vi "NameCheck.vi"(8 "error in (no error)":errorcluster, 10 "Name":string, 11 "VariableManager in":refnum<class "VariableManager.lvclass">) -> (0 "error out":errorcluster, 1 "UsedAsSequenceIndex":bool, 2 "UsedAsVariable":bool, 3 "VariableManager out":refnum<class "VariableManager.lvclass">)   [LabVIEW 2013, in "VariableManager.lvclass"]
doc: "Check the given Name agains database if it is used as a variable name or as a sequence index name (<B>idx</B>, <B>idx_f</B>, <B>idx_max</B>)."
uses:
  VariableManager.lvclass
  SequenceIndex/SequenceIndex.lvclass
  Variable/Variable.lvclass
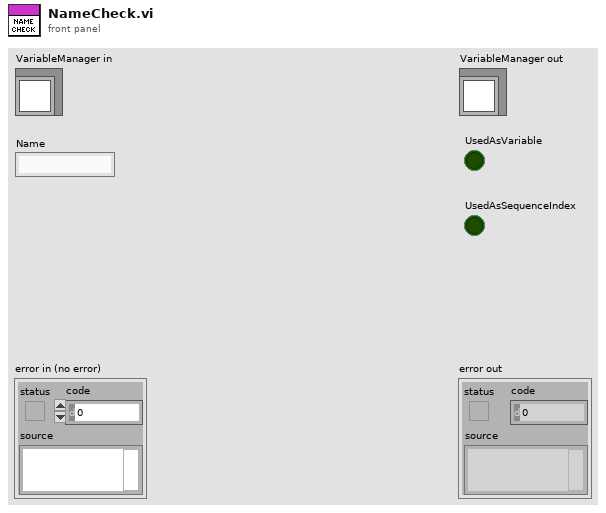
[diagram p1: front panel]
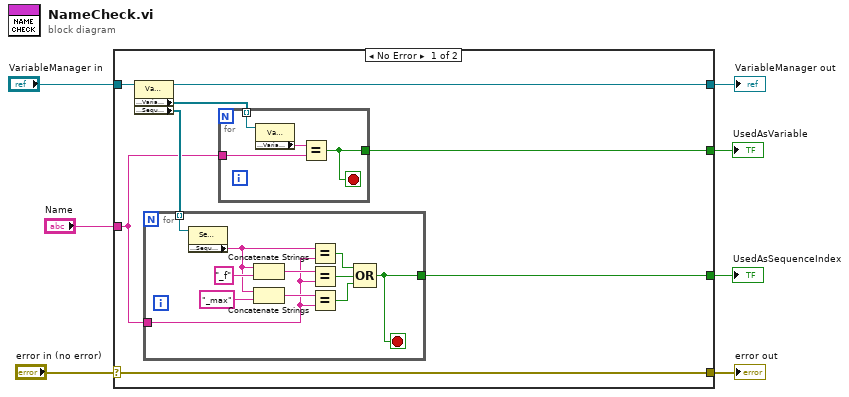
[diagram p0: block diagram]
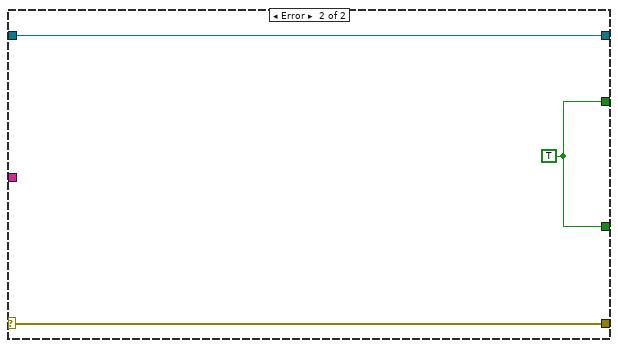
[diagram p2: hidden frame]
diagram:
  n1 = case shown="No Error" "error in (no error)" {
    selector: "error in (no error)" -> [w14 w33]
    tunnel: [w14 w33] -> w6
    tunnel: [w15 w32] -> w4
    tunnel: "VariableManager in" -> [w13 w32]
    tunnel: [w12 w31] -> w3
    tunnel: "Name" -> [w9 _]
    tunnel: [w8 w31] -> w1
    frame No Error {
      n2 = property class="VariableManager.lvclass"(reference=w13) -> (reference out=w15:refnum<class "VariableManager.lvclass">, "Accessors:Variables"=w10:refnum<class "Variable.lvclass">[], "Accessors:SequenceIndices"=w11:refnum<class "SequenceIndex.lvclass">[])  [unwired: 1 in, 1 out]
      n3 = for {
        tunnel: w11 -> [w30] mode=indexing
        tunnel: w9 -> [w24]
        tunnel: [w20] -> w12
        stop <- w20 stop-if-true
        n4 = property class="SequenceIndex.lvclass"(reference=w30) -> ("Accessors:SequenceIndexName"=w27:string)  [unwired: 1 in, 2 out]
        n5 = Concatenate Strings(w27, "_f") -> (w26:string)
        n6 = Concatenate Strings(w27, "_max") -> (w25:string)
        n7 = Equal?(x=w27, y=w24) -> (x = y?=w23:bool)
        n8 = Equal?(x=w26, y=w24) -> (x = y?=w22:bool)
        n9 = Equal?(x=w25, y=w24) -> (x = y?=w21:bool)
        n10 = Compound Arithmetic op=OR(w23, w22, w21) -> (w20:bool)
      }
      n11 = for {
        tunnel: w10 -> [w19] mode=indexing
        tunnel: w9 -> [w17]
        tunnel: [w16] -> w8
        stop <- w16 stop-if-true
        n12 = property class="Variable.lvclass"(reference=w19) -> ("Accessors:VariableName"=w18:string)  [unwired: 1 in, 2 out]
        n13 = Equal?(x=w18, y=w17) -> (x = y?=w16:bool)
      }
    }
    frame Error {
      w31 = TRUE
    }
  }
  "error out" <- w6
  "VariableManager out" <- w4
  "UsedAsSequenceIndex" <- w3
  "UsedAsVariable" <- w1
